vi "LTVUnicycleCtrl_New.vi"(9 "dT":dbl=0.02, 10 "RELMS":T2=[[0.0], [0.0]], 11 "QELMS":T2=[[0.0], [0.0], [0.0]]) -> (0 "Error":bool, 3 "LTV_UNICYCLE_CONTROLLER":T1={"m_A"=[], "m_B"=[], "m_Q"=[], "m_R"=[], "States"=0, "Inputs"=0, "PoseError"={"TRANSLATION"={"X"=0.0, "Y"=0.0}, "ROTATION"={"VALUE"=0.0, "COS"=1.0, "SIN"=0.0}}, "PoseTolerance"={"TRANSLATION"={"X"=0.0, "Y"=0.0}, "ROTATION"={"VALUE"=0.0, "COS"=1.0, "SIN"=0.0}}, "Dt"=0.02, "Enabled"=FALSE, "savedLQR_K"={"Table Xs"=[], "Table Ys"=[], "MinX"=0.0, "MaxX"=0.0, "ItemCount"=0, "Rows"=0, "Columns"=0}} {"PoseTolerance"."ROTATION"."SIN" format="%13.4f"; "PoseTolerance"."ROTATION"."COS" format="%13.4f"; "PoseTolerance"."ROTATION"."VALUE" format="%13.4f"; "PoseTolerance"."TRANSLATION"."Y" format="%14.3f"; "PoseTolerance"."TRANSLATION"."X" format="%14.3f"; "PoseError"."ROTATION"."SIN" format="%13.4f"; "PoseError"."ROTATION"."COS" format="%13.4f"; "PoseError"."ROTATION"."VALUE" format="%13.4f"; "PoseError"."TRANSLATION"."Y" format="%14.3f"; "PoseError"."TRANSLATION"."X" format="%14.3f"})   [LabVIEW 2019, in "Trajectory_Library.lvlib"]
doc: "Create implicit model follower\n\nInputs:\n - A < states, states > -- Continuous system matrix of the plant being controlled.\n - B < states, inputs > -- Continuous input matrix of the plant being controlled.\n - A_Ref < states, states > -- Continuous system matrix whose dymanics should be followed.\n - B_Ref < states, inputs > -- Continuous input matrix x whose dymanics should be followed.\n\nOutputs:\n - Error -- If TRUE, an error occured."
uses:
  Trajectory_Library.lvlib
  <vilib>/Analysis/Matrix/Datatypes/RealMatrix.ctl
  LTV_UNICYCLE_CONTROLLER.ctl
  POSE2D.ctl
  TRANSLATION2D.ctl
  ROTATION2D.ctl
  FUNCTION_GENERATOR_MATRIX.ctl
  LTV_UNICYCLE_CONTROLLER_STATE_ENUM.ctl
  Rotation_CreateAngle.vi
  Translation_Create.vi
  MatrixHelper_CoerceSize.vi
  <vilib>/gmath/interp.llb/Search Ordered Table.vi
  <vilib>/Analysis/Matrix/NI_Matrix.lvlib
panel:
  # "<3,1>"
  # "<2, 1>"
  # "<States,States>"
  # "<States,Inputs>"
  # "<States, States>"
  # "<Inputs, Inputs>"
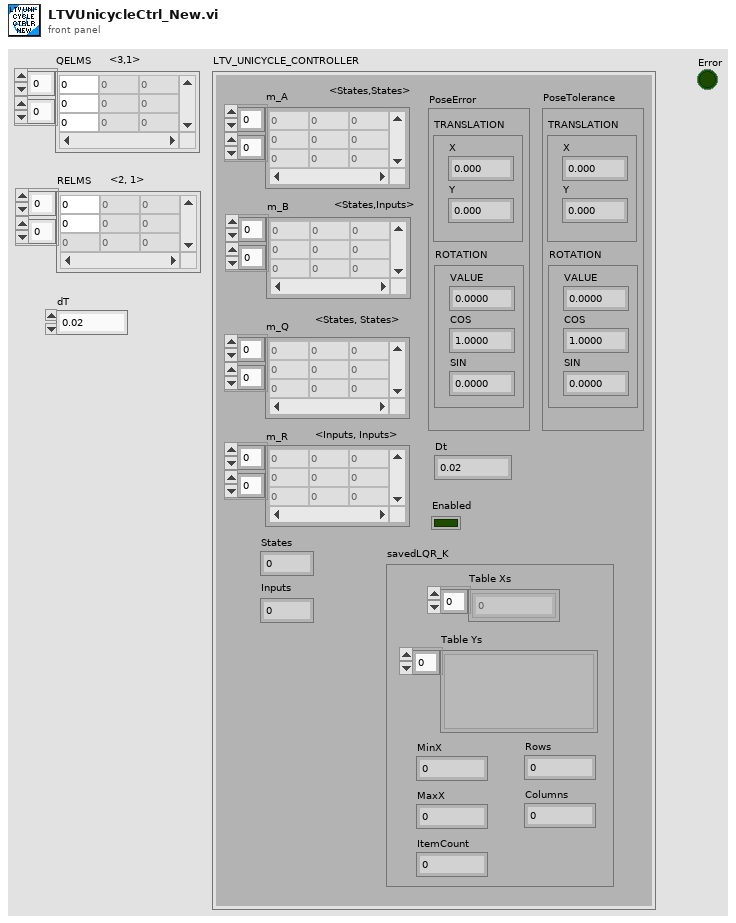
[diagram p1: front panel]
types:
  T1 = typedef "Trajectory_Library.lvlib/LTV_UNICYCLE_CONTROLLER.ctl" = cluster{"m_A":T2, "m_B":T2, "m_Q":T2, "m_R":T2, "States":i32, "Inputs":i32, "PoseError":T3, "PoseTolerance":T3, "Dt":dbl, "Enabled":bool, "savedLQR_K":T6}
  T2 = typedef "NI_Matrix.lvlib/RealMatrix.ctl" = dbl[][]
  T3 = typedef "Trajectory_Library.lvlib/POSE2D.ctl" = cluster{"TRANSLATION":T4, "ROTATION":T5}
  T4 = typedef "Trajectory_Library.lvlib/TRANSLATION2D.ctl" = cluster{"X":dbl, "Y":dbl}
  T5 = typedef "Trajectory_Library.lvlib/ROTATION2D.ctl" = cluster{"VALUE":dbl, "COS":dbl, "SIN":dbl}
  T6 = typedef "Trajectory_Library.lvlib/FUNCTION_GENERATOR_MATRIX.ctl" = cluster{"Table Xs":dbl[], "Table Ys":variant[], "MinX":dbl, "MaxX":dbl, "ItemCount":i32, "Rows":i32, "Columns":i32}
  T7 = typedef "Trajectory_Library.lvlib/LTV_UNICYCLE_CONTROLLER_STATE_ENUM.ctl" = enum16{"X", "Y", "HEADING"}
  T8 = typedef "Trajectory_Library.lvlib/LINEAR_QUADRATIC_REGULATOR.ctl" = cluster{"m_r":T2, "m_U":T2, "m_K":T2, "States":i32, "Inputs":i32}
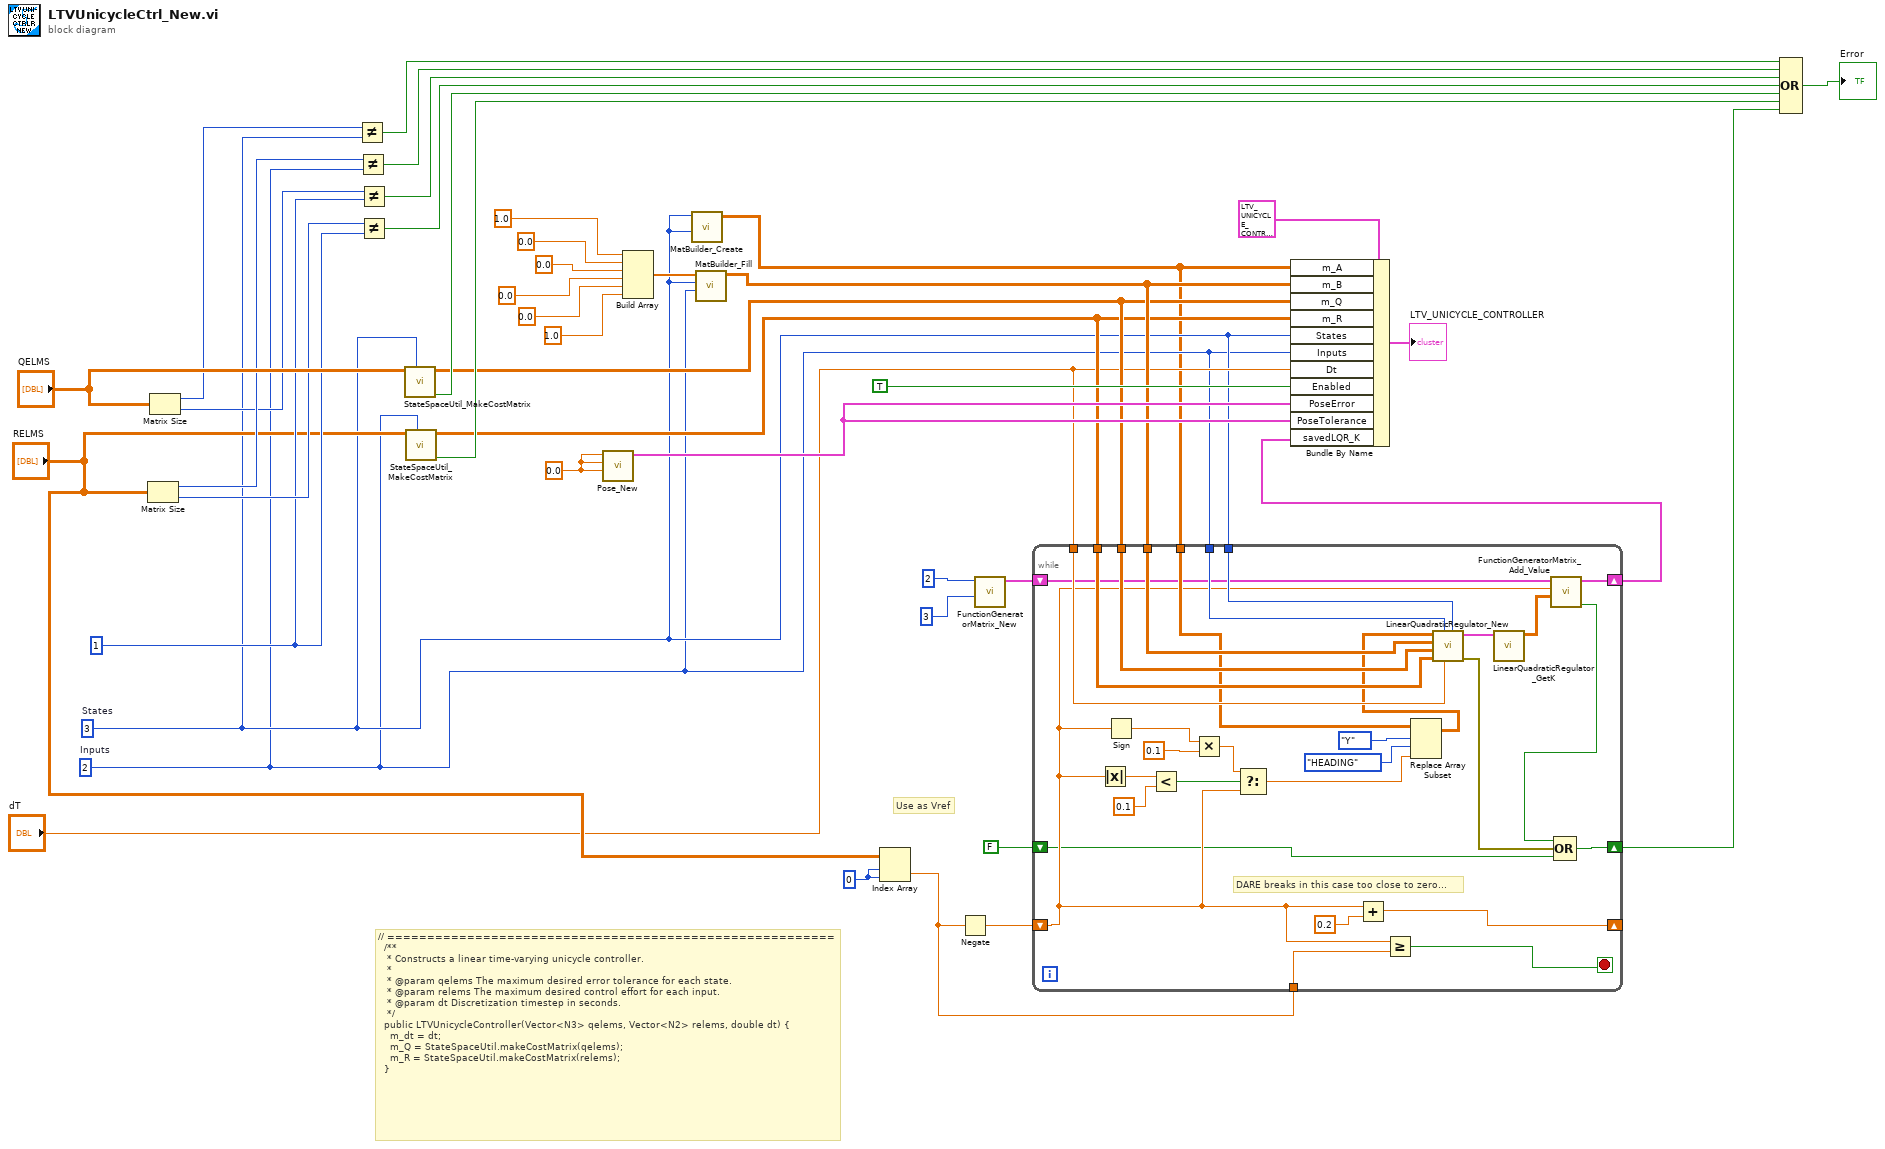
[diagram p0: block diagram]
diagram:
  w17 = 0 ("index (row)")
  w19 = 0.0 ("X")
  w7 = 2  # Inputs
  w8 = 3  # States
  w30 = 1 ("Columns")
  # "Use as Vref"
  # "// ========================================================\n  /**\n   * Constructs a linear time-varying unicycle controller.\n   *\n   * @param qelems The maximum desired error tolerance for each state.\n   * @param relems The maximum desired control effort for each input.\n   * @param dt Discretization timestep in seconds.\n   */\n  public LTVUnicycleController(Vector<N3> qelems, Vector<N2> relems, double dt) {\n    m_dt = dt;\n    m_Q = StateSpaceUtil.makeCostMatrix(qelems);\n    m_R = StateSpaceUtil.makeCostMatrix(relems);\n  }"
  n1 = Matrix Size(0:"RELMS") -> (1:w33:i32, 2:w31:i32)
  n2 = Matrix Size(0:"QELMS") -> (1:w34:i32, 2:w32:i32)
  n3 = Not Equal?(x=w34, y=w8) -> (x != y?=w42:bool)
  n4 = Not Equal?(x=w33, y=w7) -> (x != y?=w40:bool)
  n5 = Not Equal?(x=w32, y=w30) -> (x != y?=w39:bool)
  n6 = Not Equal?(x=w31, y=w30) -> (x != y?=w38:bool)
  n7 = call "StateSpaceUtil_MakeCostMatrix.vi"("Elements"=w8, "Costs"="QELMS") -> ("Sze Coerced"=w29:bool, "Costs Matrix"=w11:T2)  [unwired: 8 in]
  n8 = call "StateSpaceUtil_MakeCostMatrix.vi"("Elements"=w7, "Costs"="RELMS") -> ("Sze Coerced"=w28:bool, "Costs Matrix"=w10:T2)  [unwired: 8 in]
  n9 = call "Pose_New.vi"("Heading"=w19, "Y"=w19, "X"=w19) -> ("out POSe"=w18:T3)  [unwired: 8 in]
  n10 = Build Array(1.0 ("element"), 0.0 ("element"), 0.0 ("element"), 0.0 ("element"), 0.0 ("element"), 1.0 ("element")) -> (w27:dbl[])
  n11 = call "MatBuilder_Create.vi"("Columns"=w8, "Rows"=w8) -> ("output matrix"=w6:T2)  [unwired: 9 in]
  n12 = call "MatBuilder_Fill.vi"("Columns"=w7, "Rows"=w8, "Value List"=w27) -> ("output matrix"=w12:T2)  [unwired: 8 in]
  n13 = Index Array(array="RELMS", index (row)=w17, index (col)=w17) -> (element=w14:dbl)
  n14 = Negate(x=w14) -> (-x=w15:dbl)
  n15 = call "FunctionGeneratorMatrix_New.vi"("Columns"=3, "Rows"=2) -> ("FUNCTION_GENERATOR_MATRIX"=w13:T6)  [unwired: 9 in]
  n16 = while {
    shift-right: [w69] -> _
    shift-left: w15 -> [w49]
    tunnel: w14 -> [w71]
    tunnel: w12 -> [w68]
    tunnel: w11 -> [w67]
    tunnel: w10 -> [w66]
    tunnel: "dT" -> [w65]
    tunnel: w8 -> [w64]
    tunnel: w7 -> [w63]
    tunnel: w6 -> [w53]
    shift-right: [w50] -> w5
    shift-left: w13 -> [w47]
    shift-right: [w45] -> w1
    shift-left: FALSE -> [w46]
    stop <- w70 stop-if-true
    # "DARE breaks in this case too close to zero..."
    n17 = Absolute Value(x=w49) -> (abs(x)=w62:dbl)
    n18 = Sign(1:w49) -> (0:w57:dbl)
    n19 = Less?(x=w62, y=0.1) -> (x < y?=w60:bool)
    n20 = Multiply(x=w57, y=0.1 ("t")) -> (x*y=w59:dbl)
    n21 = Select(t=w59, s=w60, f=w49) -> (s? t:f=w54:dbl)
    n22 = Add(x=w49, y=0.2) -> (x+y=w69:dbl)
    n23 = Greater Or Equal?(x=w49, y=w71) -> (x >= y?=w70:bool)
    n24 = Replace Array Subset(array=w53, new element=w54, index (row)=LTV_UNICYCLE_CONTROLLER_STATE_ENUM."Y" ("LTV_UNICYCLE_CONTROLLER_STATE"), index (col)=LTV_UNICYCLE_CONTROLLER_STATE_ENUM."HEADING" ("LTV_UNICYCLE_CONTROLLER_STATE")) -> (w52:T2)
    n25 = call "LinearQuadraticRegulator_New.vi"("States"=w64, "dt_Seconds"=w65, "Inputs"=w63, "R"=w66, "Q"=w67, "B"=w68, "A"=w52) -> ("Error"=w44:errorcluster, "LinearQuadraticRegulator"=w51:T8)  [unwired: 3 in]
    n26 = call "LinearQuadraticRegulator_GetK.vi"("in LinearQuadraticRegulator"=w51) -> ("K"=w48:T2)  [unwired: 10 in]
    n27 = call "FunctionGeneratorMatrix_Add_Value.vi"("Y Value"=w48, "X Value"=w49, "in FUNC_GEN_MATRIX"=w47) -> ("Error"=w43:bool, "out FUNC_GEN_MATRIX"=w50:T6)  [unwired: 7 in]
    n28 = Compound Arithmetic op=OR(w43, w44, w46) -> (w45:bool)
  }
  n29 = Bundle By Name(cluster=T1 {"m_A"=[], "m_B"=[], "m_Q"=[], "m_R"=[], "States"=0, "Inputs"=0, "PoseError"={"TRANSLATION"={"X"=0.0, "Y"=0.0}, "ROTATION"={"VALUE"=0.0, "COS"=1.0, "SIN"=0.0}}, "PoseTolerance"={"TRANSLATION"={"X"=0.0, "Y"=0.0}, "ROTATION"={"VALUE"=0.0, "COS"=1.0, "SIN"=0.0}}, "Dt"=0.02, "Enabled"=FALSE, "savedLQR_K"={"Table Xs"=[], "Table Ys"=[], "MinX"=0.0, "MaxX"=0.0, "ItemCount"=0, "Rows"=0, "Columns"=0}} ("LTV_UNICYCLE_CONTROLLER"), "m_A"=w6, "m_B"=w12, "m_Q"=w11, "m_R"=w10, "States"=w8, "Inputs"=w7, "Dt"="dT", "Enabled"=TRUE, "PoseError"=w18, "PoseTolerance"=w18, "savedLQR_K"=w5) -> (→"LTV_UNICYCLE_CONTROLLER":T1)
  n30 = Compound Arithmetic op=OR(w42, w40, w39, w38, w29, w28, w1) -> (→"Error":bool)
